vi "FormulaNode.vi"() -> ()   [LabVIEW 2020]
panel:
  out "y":i32
  in  "x":dbl
  # "Formual Node"
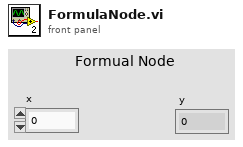
[diagram p1: front panel]
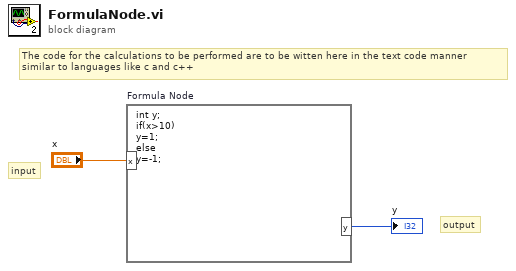
[diagram p0: block diagram]
diagram:
  # "input"
  # "output"
  # "The code for the calculations to be performed are to be witten here in the text code manner \nsimilar to languages like c and c++"
  n1 = formula code="int y;\nif(x>10)\ny=1;\nelse \ny=-1;"("x"="x") -> ("y"=→"y":i32)
